vi "CLD 17 Number Pad Solution Two.vi"() -> ()   [LabVIEW 2009]
doc: "CLD 17\n\nThis VI uses an event structure to respond to changes in the GUI."
uses:
  CLD 17 Keypad_Typedef.ctl
panel:
  out "String":string="0"
  out "Numeric":dbl
  in  "Keypad Cluster":T1
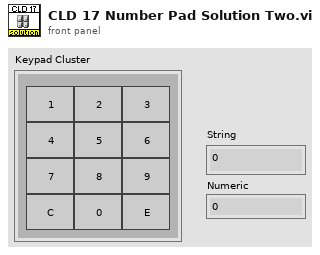
[diagram p1: front panel]
types:
  T1 = typedef "CLD 17 Keypad_Typedef.ctl" = cluster{"0":bool, "1":bool, "2":bool, "3":bool, "4":bool, "5":bool, "6":bool, "7":bool, "8":bool, "9":bool, "C":bool, "E":bool}
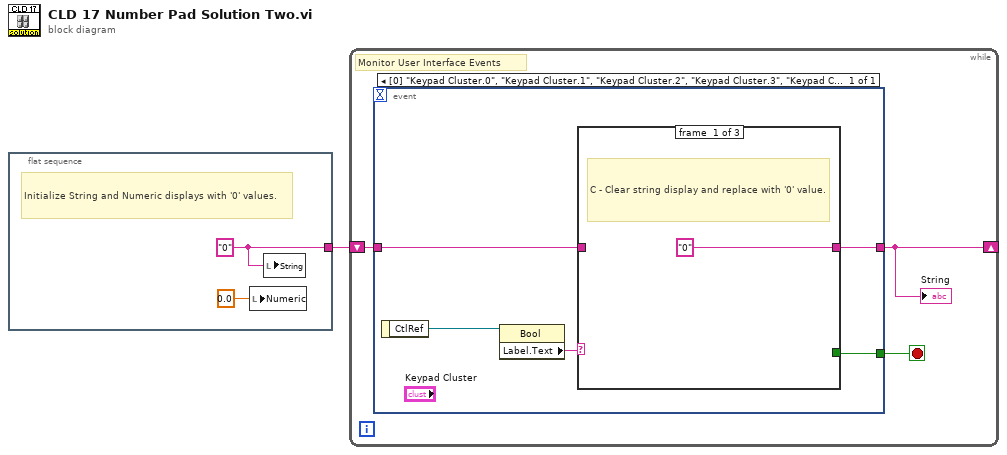
[diagram p0: block diagram]
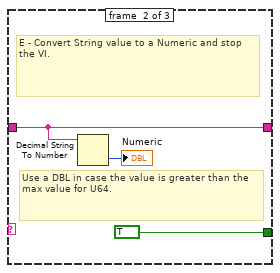
[diagram p2: hidden frame]
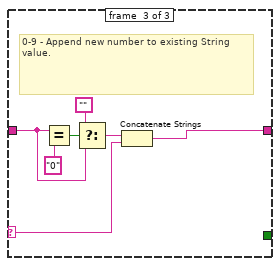
[diagram p3: hidden frame]
diagram:
  n1 = flat-sequence {
    tunnel: [w3] -> w1
    frame #0 {
      w3 = "0" ("Current String Value")
      # "Initialize String and Numeric displays with '0' values."
      n2 = local write "Numeric"(0.0 ("Numeric")) -> ()
      n3 = local write "String"(w3) -> ()
    }
  }
  n4 = while {
    shift-right: [w4] -> _
    shift-left: w1 -> [w5]
    stop <- w6 stop-if-true
    # "Monitor User Interface Events"
    n5 = event shown="[0] \"Keypad Cluster.0\", \"Keypad Cluster.1\", \"Keypad Cluster.2\", \"Keypad Cluster.3\", \"Keypad Cluster.4\", \"Keypad Cluster.5\", \"Keypad Cluster.6\", \"Keypad Cluster.7\", \"Keypad Cluster.8\", \"Keypad Cluster.9\", \"Keypad Cluster.C\", \"Keypad Cluster.E\": Value Change" {
      selector: _ -> [_]
      dyn-events: _ -> [_]
      timeout: _ -> [_]
      tunnel: [w7] -> w6
      tunnel: w5 -> [w10]
      tunnel: [w9] -> w4
      event [0] "Keypad Cluster.0", "Keypad Cluster.1", "Keypad Cluster.2", "Keypad Cluster.3", "Keypad Cluster.4", "Keypad Cluster.5", "Keypad Cluster.6", "Keypad Cluster.7", "Keypad Cluster.8", "Keypad Cluster.9", "Keypad Cluster.C", "Keypad Cluster.E": Value Change {
        # "0-9 - Append new number to existing String value."
        n6 = event-data() -> ("CtlRef"=w11:refnum<vi>)  [unwired: 1 in]
        n7 = property class="Bool"(reference=w11) -> ("Label.Text"=w8:string)  [unwired: 1 in, 2 out]
        n8 = case shown="\"E\"" w8 {
          selector: w8 -> [_ _ w16]
          tunnel: w10 -> [_ w13 w19]
          tunnel: ["0" ("Current String Value") w13 w17] -> w9
          tunnel: [_ TRUE _] -> w7
          frame #0 {
            # "C - Clear string display and replace with '0' value."
          }
          frame #1 {
            # "Use a DBL in case the value is greater than the max value for U64."
            # "E - Convert String value to a Numeric and stop the VI."
            n9 = Decimal String To Number(string=w13) -> (number=→"Numeric":i32)  [unwired: 2 in, 1 out]
          }
          frame #2 {
            # "0-9 - Append new number to existing String value."
            n10 = Equal?(x=w19, y="0" ("Current String Value")) -> (x = y?=w21:bool)
            n11 = Select(t="", s=w21, f=w19) -> (s? t:f=w18:string)
            n12 = Concatenate Strings(w18, w16) -> (w17:string)
          }
        }
      }
    }
    "String" <- w4
  }
